vi "getNamesFromPath.vi"(4 "error in (no error)":errorcluster, 7 "tree path":string) -> (0 "error out":errorcluster, 2 "channel":string, 3 "group":string)   [LabVIEW 2018]
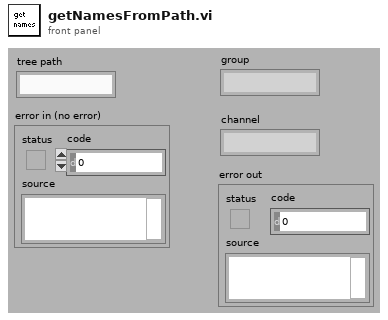
[diagram p1: front panel]
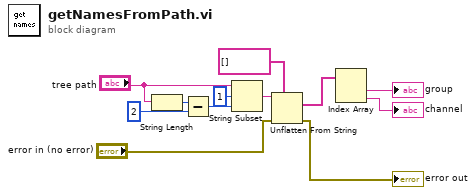
[diagram p0: block diagram]
diagram:
  n1 = String Length(string="tree path") -> (length=w6:i32)
  n2 = Subtract(x=w6, y=2 ("offset (0)")) -> (x-y=w8:i32)
  n3 = String Subset(string="tree path", offset (0)=1, length (rest)=w8) -> (substring=w9:string)
  n4 = Unflatten From String(type=string[] [], binary string=w9, error in (no error)="error in (no error)") -> (value=w2:string[], error out=→"error out":errorcluster)  [unwired: 2 in, 1 out]
  n5 = Index Array(array=w2) -> (element #1=→"group":string, element #2=→"channel":string)  [unwired: 2 in]
